vi "Change Bookmarks Grouping.vi"(8 "Error In":errorcluster, 9 "Data":variant, 10 "Messages In":refnum<queue>, 11 "State In":T1) -> (0 "Error Out":errorcluster, 2 "Messages Out":refnum<queue>, 3 "State Out":T1)   [LabVIEW 2018, in "Bookmark Manager.lvlib"]
uses:
  Bookmark Manager.lvlib
  Controls/State.ctl
  <vilib>/addons/analyzer/_analyzerctrls.llb/VIAnCtl Analysis App Info.ctl
  Controls/Bookmark.ctl
  Controls/VI Identifier.ctl
  Controls/Bookmarks Groups.ctl
  Controls/Message.ctl
  Parameter Keys.vi
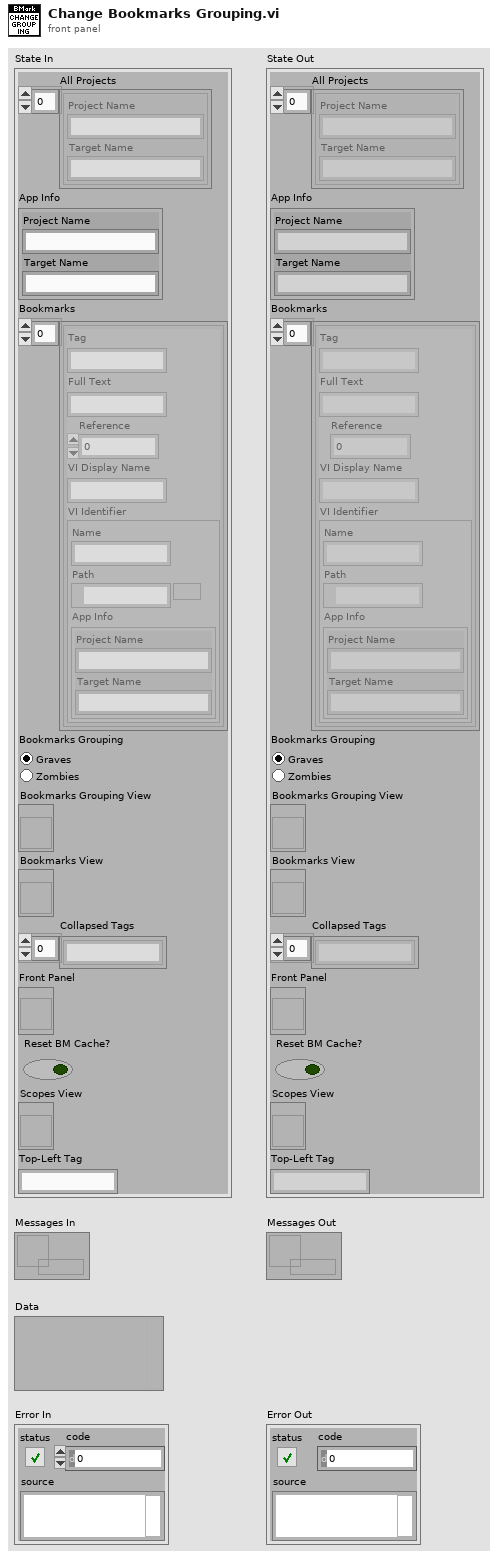
[diagram p1: front panel]
types:
  T1 = typedef "Bookmark Manager.lvlib/State.ctl" = cluster{"All Projects":T2[], "App Info":T2, "Bookmarks":T3[], "Bookmarks Grouping":T5, "Bookmarks Grouping View":refnum<vi>, "Bookmarks View":refnum<vi>, "Collapsed Tags":string[], "Front Panel":refnum<vi>, "Reset BM Cache?":bool, "Scopes View":refnum<vi>, "Top-Left Tag":string}
  T2 = typedef "VIAnCtl Analysis App Info.ctl" = cluster{"Project Name":string, "Target Name":string}
  T3 = typedef "Bookmark Manager.lvlib/Bookmark.ctl" = cluster{"Tag":string, "Full Text":string, "Reference":i32, "VI Display Name":string, "VI Identifier":T4}
  T4 = typedef "Bookmark Manager.lvlib/VI Identifier.ctl" = cluster{"Name":string, "Path":path, "App Info":T2}
  T5 = typedef "Bookmark Manager.lvlib/Bookmarks Groups.ctl" = enum32{"Graves", "Zombies"}
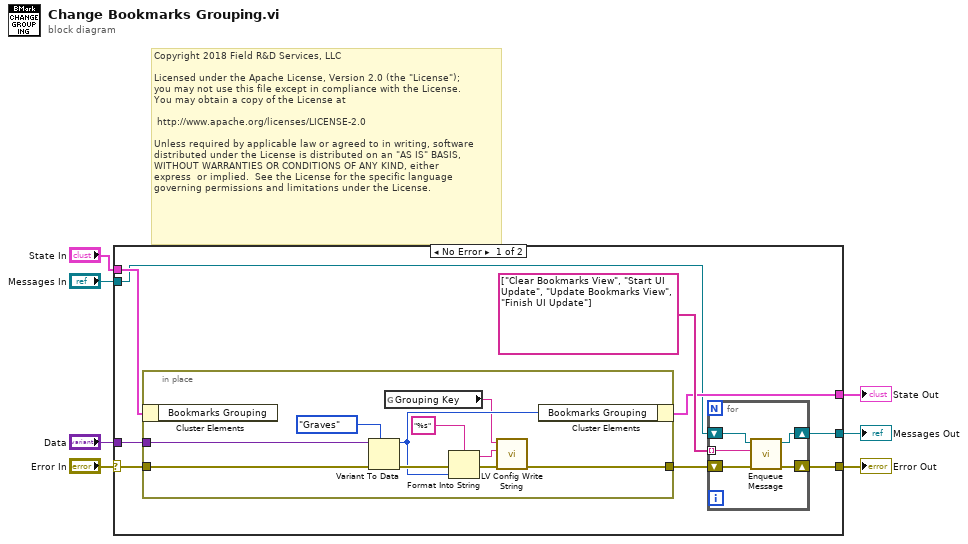
[diagram p0: block diagram]
diagram:
  # "Copyright 2018 Field R&D Services, LLC\n\nLicensed under the Apache License, Version 2.0 (the \"License\");\nyou may not use this file except in compliance with the License.\nYou may obtain a copy of the License at\n\n\thttp://www.apache.org/licenses/LICENSE-2.0\n\nUnless required by applicable law or agreed to in writing, software\ndistributed under the License is distributed on an \"AS IS\" BASIS,\nWITHOUT WARRANTIES OR CONDITIONS OF ANY KIND, either \nexpress  or implied.  See the License for the specific language \ngoverning permissions and limitations under the License."
  n1 = case shown="No Error" "Error In" {
    selector: "Error In" -> [w10 w33]
    tunnel: [w15 w33] -> w7
    tunnel: [w13 w34] -> w6
    tunnel: "State In" -> [w12 w34]
    tunnel: "Data" -> [w11 _]
    tunnel: "Messages In" -> [w9 w32]
    tunnel: [w8 w32] -> w1
    frame No Error {
      n2 = in-place {
        in-place-border: w10 -> [w31]
        in-place-border: [w27] -> w14
        in-place-border: w11 -> [w30]
        n3 = in-place-cluster #1(w12) -> ()  [unwired: 1 out]
        n4 = Variant To Data(error in=w31, type=Bookmarks_Groups."Graves" ("Bookmarks Filter"), Variant=w30) -> (data=w24:T5, error out=w28:errorcluster)
        n5 = global read "Parameter Keys.vi" "Grouping Key"() -> (w22:string)
        n6 = Format Into String(format string="%s", error in=w28, w24) -> (resulting string=w23:string, error out=w26:errorcluster)  [unwired: 1 in]
        n7 = call <resource>:"LV Config Write String.vi"("error in (no error)"=w26, "value"=w23, "key"=w22) -> ("error out"=w27:errorcluster)  [unwired: 4 in]
        n8 = in-place-cluster #1("Bookmarks Grouping"=w24) -> (w13:T1)
      }
      n9 = for {
        shift-right: [w20] -> w15
        shift-left: w14 -> [w21]
        tunnel: string[] ["Clear Bookmarks View", "Start UI Update", "Update Bookmarks View", "Finish UI Update"] -> [w19] mode=indexing
        shift-right: [w17] -> w8
        shift-left: w9 -> [w18]
        n10 = call "Enqueue Message.vi"("Error In"=w21, "Command"=w19, "Message Queue In"=w18) -> ("Error Out"=w20:errorcluster, "Message Queue Out"=w17:refnum<queue>)  [unwired: 7 in]
      }
    }
    frame Error {
    }
  }
  "Error Out" <- w7
  "State Out" <- w6
  "Messages Out" <- w1
